vi "Configure Automatic Discharge.vi"(8 "error in (no error)":errorcluster, 9 "Discharge Level (2.000000E-6)":dbl=2e-06 format="%.6e", 10 "Auto Discharge (F: Disable)":bool, 11 "VISA resource name":refnum<visa-resource-name>) -> (0 "error out":errorcluster, 3 "VISA resource name out":refnum<visa-resource-name>)   [LabVIEW 2016, in "Keithley 6517.lvlib"]
doc: "Controls the auto discharge state and configures the discharge level for coulombs."
uses:
  <instrlib>/Keithley 6517/Keithley 6517.lvlib
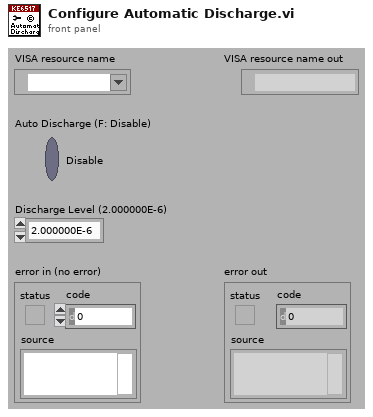
[diagram p1: front panel]
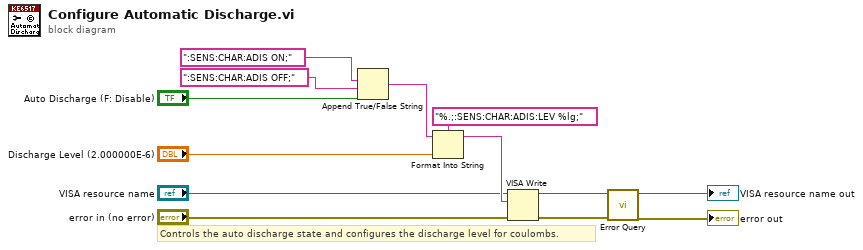
[diagram p0: block diagram]
diagram:
  # "Controls the auto discharge state and configures the discharge level for coulombs."
  n1 = Append True/False String(1:"Auto Discharge (F: Disable)", 2:":SENS:CHAR:ADIS OFF;", 3:":SENS:CHAR:ADIS ON;") -> (0:w10:string)  [unwired: 1 in]
  n2 = Format Into String(format string="%.;:SENS:CHAR:ADIS:LEV %lg;", initial string=w10, "Discharge Level (2.000000E-6)") -> (resulting string=w7:string)  [unwired: 1 in, 1 out]
  n3 = VISA Write(VISA resource name="VISA resource name", write buffer=w7, error in (no error)="error in (no error)") -> (VISA resource name out=w5:refnum<visa-resource-name>, error out=w4:errorcluster)  [unwired: 1 out]
  n4 = call <instrlib>:"Error Query.vi"("error in (no error)"=w4, "VISA resource name"=w5) -> ("error out"=→"error out":errorcluster, "VISA resource name out"=→"VISA resource name out":refnum<visa-resource-name>)  [unwired: 6 in, 2 out]
